vi "run.get.vi"(8 "error in":errorcluster, 10 "Run RID":string, 11 "Nominal Client in":refnum<class "Nominal Client.lvclass">) -> (0 "error out":errorcluster, 2 "Run":refnum<class "Run.lvclass">, 3 "Nominal Client out":refnum<class "Nominal Client.lvclass">)   [LabVIEW 2020, in "Nominal Client.lvclass"]
doc: "Fetches details about the run in question based on its RID."
uses:
  Nominal Client.lvclass
  Run/Run.lvclass
  Nominal Client.lvclass/Nominal Client.ctl
  create.authorization_header.vi
  trace.payload_sent.vi
  trace.payload_received.vi
  error.vi
  api_token.get.vi
  trace.calling_method.vi
  <vilib>/JDP Science/JDP Science Common Utilities/Trim Whitespace__JDP.vi
  <vilib>/AdvancedString/1D String Array to Delimited String.vi
  error.vi/859f8e04-e495-489b-b5b4-7ac163f56130.vi
  <vilib>/Utility/libraryn.llb/Get File Extension.vi
  log_file.write.vi
  <vilib>/JDP Science/JSONtext/Get all Object Items.vi
  <vilib>/Utility/error.llb/Error Cluster From Error Code.vi
  <vilib>/JDP Science/JSONtext/JSON text to Variant.vi
  <vilib>/JDP Science/JSONtext/LVClass Serializer/JSONtext LVClass Serializer.lvclass
  <vilib>/addons/_JKI.lib/REST Client/classes/Response Headers/Response Headers.lvclass
  <vilib>/addons/_JKI.lib/REST Client/classes/REST Client/REST Client.lvclass
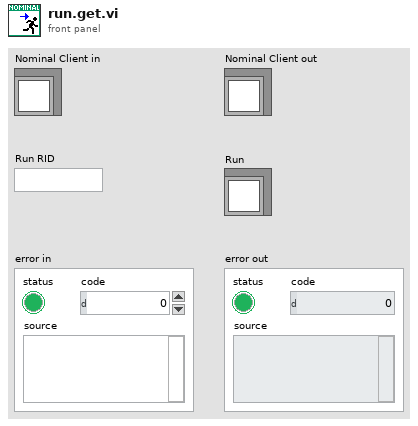
[diagram p1: front panel]
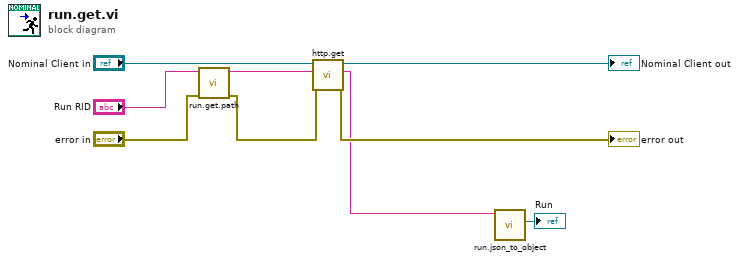
[diagram p0: block diagram]
diagram:
  n1 = call "run.get.path.vi"("error in"="error in", "Run RID"="Run RID") -> ("error out"=w5:errorcluster, "pah"=w6:string)  [unwired: 8 in]
  n2 = call "http.get.vi"("error in"=w5, "Path"=w6, "Nominal Client in"="Nominal Client in") -> ("error out"=→"error out":errorcluster, "Response"=w2:string, "Nominal Client out"=→"Nominal Client out":refnum<class "Nominal Client.lvclass">)  [unwired: 5 in, 1 out]
  n3 = call "run.json_to_object.vi"("JSON"=w2) -> ("Run"=→"Run":refnum<class "Run.lvclass">)  [unwired: 9 in, 1 out]
